vi "Timer.vi"(8 "error out":errorcluster) -> (0 "errout":errorcluster caption="sortie d'erreur", 4 "30s?":bool)   [LabVIEW 2020]
uses:
  VG/VG_progressBar.vi
panel:
  out "Chargement":u8(slide) scale=0.0..30.0
  out "Chaîne":string="dzdz"
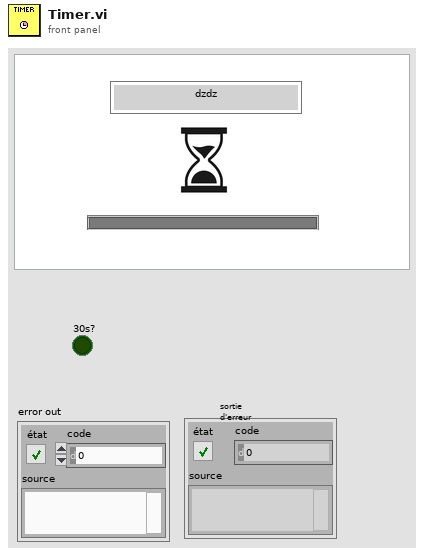
[diagram p1: front panel]
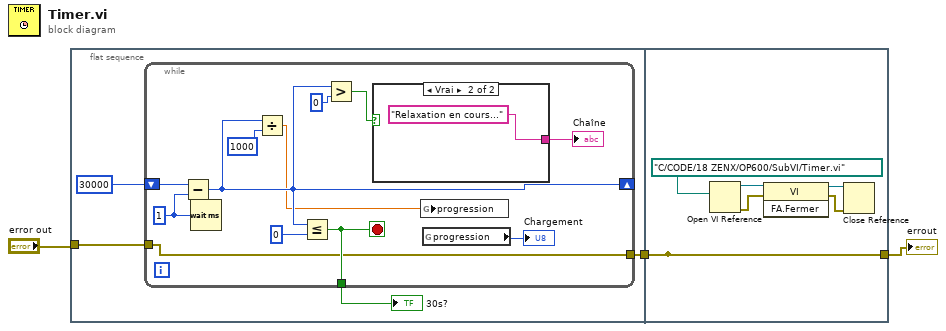
[diagram p0: block diagram]
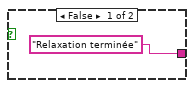
[diagram p2: hidden frame]
diagram:
  n1 = flat-sequence {
    tunnel: "error out" -> [w5]
    tunnel: [w4] -> w3
    tunnel: [w22] -> _
    tunnel: w3 -> [w22]
    tunnel: [w22] -> w2
    frame #0 {
      n2 = while {
        shift-right: [w15] -> _
        shift-left: u32 30000 ("attente (ms)") -> [w19]
        tunnel: [w11] -> w6
        tunnel: w5 -> [w8]
        tunnel: [w8] -> w4
        stop <- w11 stop-if-true
        w17 = u32 1 ("attente (ms)")
        n3 = Subtract(x=w19, y=w17) -> (x-y=w15:u32)
        n4 = Wait (ms)(milliseconds to wait=w17) -> ()  [unwired: 1 out]
        n5 = Divide(x=w15, y=u32 1000) -> (x/y=w10:dbl)
        n6 = Less Or Equal?(x=w15, y=u32 0) -> (x <= y?=w11:bool)
        n7 = Greater?(x=w15, y=u32 0) -> (0:w13:bool)
        n8 = case shown="Vrai" w13 {
          tunnel: ["Relaxation terminée" "Relaxation en cours..."] -> w12
          frame False {
          }
          frame True {
          }
        }
        "Chaîne" <- w12
        n9 = global write "VG_progressBar.vi" "progression"(w10) -> ()
        n10 = global read "VG_progressBar.vi" "progression"() -> (→"Chargement":u8)
      }
      "30s?" <- w6
    }
    frame #1 {
      n11 = Open VI Reference(vi path=path "C:/CODE/18 ZENX/OP600/SubVI/Timer.vi" ("chemin du VI")) -> (vi reference=w24:refnum<vi>, error out=w27:errorcluster)  [unwired: 5 in]
      n12 = invoke class="VI" method="FA.Fermer"(reference=w24, error in=w27) -> (reference out=w26:refnum<vi>, error out=w25:errorcluster)  [unwired: 1 in, 1 out]
      n13 = Close Reference(reference=w26, error in (no error)=w25) -> ()  [unwired: 1 out]
    }
  }
  "errout" <- w2
